vi "Folder_Create Menu Element.vi"(7 "Run Data":T1={"Target Folder"=path "", "Menu Folder"=path "", "Active Folder"=path "", "Config"={"Main"={"Menu Folder"="", "Re-Create Menu Folder?"=FALSE, "Allow mnu replace?"=FALSE, "Relative Link Target"=""}, "File Filter"={"Exclude Prefixes"=[], "Ignore Names"=[], "Include Extensions"=[], "Exclude Postfixes"=[]}, "Folder Filter"={"Exclude Prefixes"=[], "Ignore Names"=[]}, "File Name Edit"={"Pre Split String"="", "Post Split String"="", "Deletion Strings"=[]}, "Folder Name Edit"={"Pre Split String"="", "Post Split String"="", "Deletion Strings"=[]}, "Folder Icon Map"={}, "Default Palette Data"={"Display Name Override"="", "View Format"=2, "Palette Width"=0, "Help Tag"="", "Help File Path"=path "", "Palette Description"=""}, "Default File Data"={"Display Name Override"="", "Place VI Contents?"=FALSE}, "Palette Override map"={}, "File Override map"={}}} {"Config"."Default Palette Data"."View Format" items=["Icons", "Text", "Icons and Text"]}, 8 "error in (no error)":errorcluster, 11 "Array in":path[](array[path])) -> (0 "error out":errorcluster, 3 "Folder Elements out":T11[](array[typedef]))   [LabVIEW 2019, in "AutoMenuCreator.lvlib"]
uses:
  AutoMenuCreator.lvlib
  <vilib>/Palette API/Palette Menu/Public Type Define/Item.ctl
  Ctl/Ctl_Run Data.ctl
  Ctl/Ctl_Config.ctl
  Ctl/Ctl_Config_Main.ctl
  Ctl/Ctl_Config_File Filter.ctl
  Ctl/Ctl_Config_Folder Filter.ctl
  Ctl/Ctl_Config_Name Edit.ctl
  Ctl/Ctl_Config_Folder Icon Map.ctl
  Ctl/Ctl_Config_Palette Data.ctl
  <vilib>/Palette API/Palette Menu/Public Type Define/View Format.ctl
  Ctl/Ctl_Config_File Data.ctl
  <vilib>/Palette API/Palette Menu/Palette Menu.lvlib
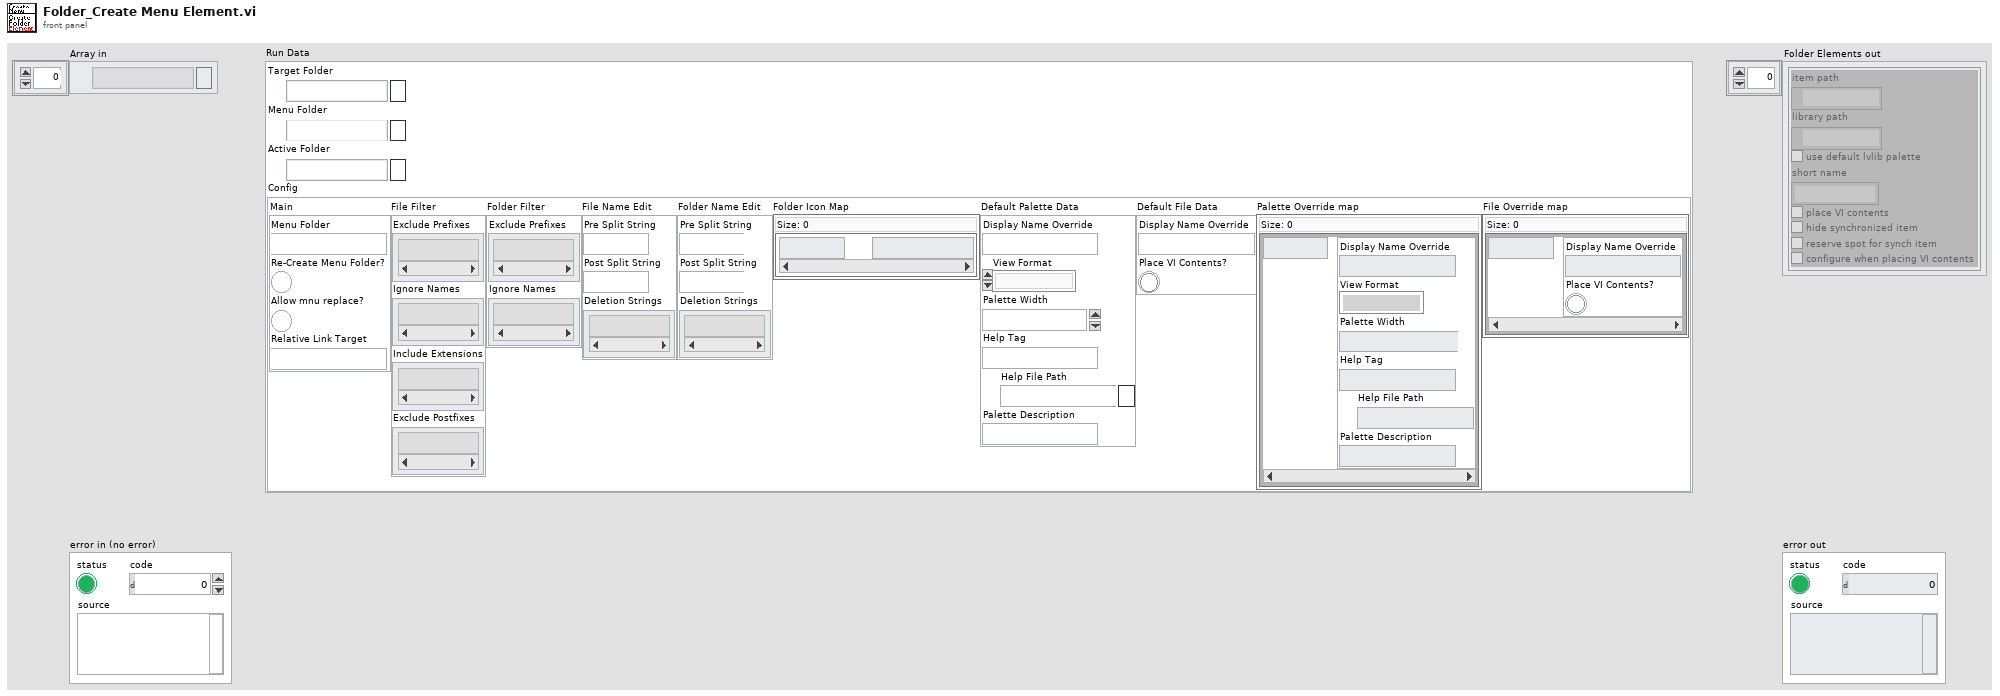
[diagram p1: front panel]
types:
  T1 = typedef "AutoMenuCreator.lvlib/Ctl_Run Data.ctl" = cluster{"Target Folder":path, "Menu Folder":path, "Active Folder":path, "Config":T2}
  T2 = typedef "AutoMenuCreator.lvlib/Ctl_Config.ctl" = cluster{"Main":T3, "File Filter":T4, "Folder Filter":T5, "File Name Edit":T6, "Folder Name Edit":T6, "Folder Icon Map":T7, "Default Palette Data":T8, "Default File Data":T10, "Palette Override map":map{string, T8}, "File Override map":map{string, T10}}
  T3 = typedef "AutoMenuCreator.lvlib/Ctl_Config_Main.ctl" = cluster{"Menu Folder":string, "Re-Create Menu Folder?":bool, "Allow mnu replace?":bool, "Relative Link Target":string}
  T4 = typedef "AutoMenuCreator.lvlib/Ctl_Config_File Filter.ctl" = cluster{"Exclude Prefixes":string[], "Ignore Names":string[], "Include Extensions":string[], "Exclude Postfixes":string[]}
  T5 = typedef "AutoMenuCreator.lvlib/Ctl_Config_Folder Filter.ctl" = cluster{"Exclude Prefixes":string[], "Ignore Names":string[]}
  T6 = typedef "AutoMenuCreator.lvlib/Ctl_Config_Name Edit.ctl" = cluster{"Pre Split String":string, "Post Split String":string, "Deletion Strings":string[]}
  T7 = typedef "AutoMenuCreator.lvlib/Ctl_Config_Folder Icon Map.ctl" = map{string, path}
  T8 = typedef "AutoMenuCreator.lvlib/Ctl_Config_Palette Data.ctl" = cluster{"Display Name Override":string, "View Format":T9, "Palette Width":i16, "Help Tag":string, "Help File Path":path, "Palette Description":string}
  T9 = typedef "Palette Menu.lvlib/View Format.ctl" = u16
  T10 = typedef "AutoMenuCreator.lvlib/Ctl_Config_File Data.ctl" = cluster{"Display Name Override":string, "Place VI Contents?":bool}
  T11 = typedef "Palette Menu.lvlib/Item.ctl" = cluster{"item path":path, "library path":path, "use default lvlib palette":bool, "short name":string, "place VI contents":bool, "hide synchronized item":bool, "reserve spot for synch item":bool, "configure when placing VI contents":bool}
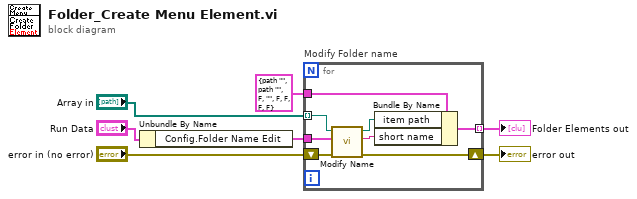
[diagram p0: block diagram]
diagram:
  n1 = Unbundle By Name("Run Data") -> ("Config.Folder Name Edit"=w1:T6)
  n2 = for "Modify Folder name" {
    tunnel: T11 {"item path"=path "", "library path"=path "", "use default lvlib palette"=FALSE, "short name"="", "place VI contents"=FALSE, "hide synchronized item"=FALSE, "reserve spot for synch item"=FALSE, "configure when placing VI contents"=FALSE} ("items") -> [w15]
    tunnel: "Array in" -> [w12] mode=indexing
    tunnel: [w14] -> w4 mode=indexing
    shift-right: [w9] -> w6
    shift-left: "error in (no error)" -> [w10]
    tunnel: w1 -> [w8]
    n3 = call "Modify Name.vi"("error in (no error)"=w10, "Name Edit Config"=w8, "Path in"=w12) -> ("error out"=w9:errorcluster, "Formatted name"=w11:string, "Dup Path out"=w13:path)  [unwired: 6 in]
    n4 = Bundle By Name(cluster=w15, "item path"=w13, "short name"=w11) -> (w14:T11)
  }
  "error out" <- w6
  "Folder Elements out" <- w4
